vi "Hello World.vi"(8 "error in (no error)":errorcluster) -> (0 "error out":errorcluster)   [LabVIEW 2010]
panel:
  in  "stop":bool
  out "Slide":u8(slide) scale=0.0..100.0
  # "Hello World!!!"
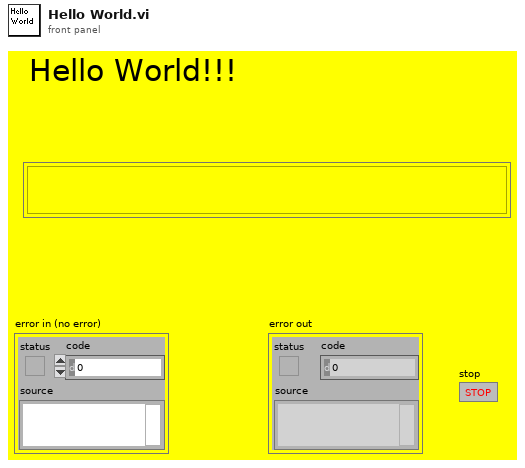
[diagram p1: front panel]
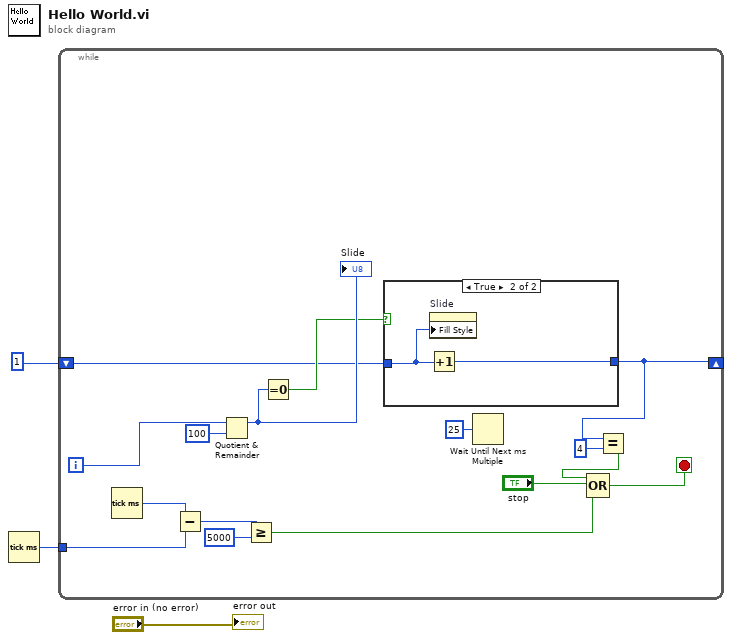
[diagram p0: block diagram]
diagram:
  n1 = Tick Count (ms)() -> (millisecond timer value=w2:u32)
  n2 = while {
    shift-right: [w6] -> _
    shift-left: 1 ("Fill Style") -> [w15]
    tunnel: w2 -> [w13]
    i -> [w7]
    stop <- w8 stop-if-true
    n3 = Tick Count (ms)() -> (millisecond timer value=w14:u32)
    n4 = Subtract(x=w14, y=w13) -> (x-y=w12:u32)
    n5 = Quotient & Remainder(x=w7, y=100) -> (x-y*floor(x/y)=w17:i32)  [unwired: 1 out]
    "Slide" <- w17
    n6 = Greater Or Equal?(x=w12, y=u32 5000) -> (x >= y?=w9:bool)
    n7 = Equal To 0?(x=w17) -> (x = 0?=w16:bool)
    n8 = case shown="True" w16 {
      tunnel: w15 -> [w20 w22]
      tunnel: [w20 w21] -> w6
      frame False {
      }
      frame True {
        n9 = Increment(x=w22) -> (x+1=w21:i32)
        n10 = property on="Slide" class="Slide (strict)"("Fill Style"=w22) -> ()  [unwired: 2 in, 2 out]
      }
    }
    n11 = Wait Until Next ms Multiple(millisecond multiple=u32 25) -> ()  [unwired: 1 out]
    n12 = Equal?(x=w6, y=4) -> (x = y?=w4:bool)
    n13 = Compound Arithmetic op=OR(w4, "stop", w9) -> (w8:bool)
  }
  "error out" <- "error in (no error)"
